vi "Serial_comm.vi"() -> ()   [LabVIEW 2022 SP3]
panel:
  in  "byte count":u32
  out "return count":u32
  out "read buffer":string
  in  "stop":bool
  in  "VISA resource name":refnum<visa-resource-name>
  # "This sets the number of digits displayed (1 digit = 1 byte) plus 2 bytes of terminating characters"
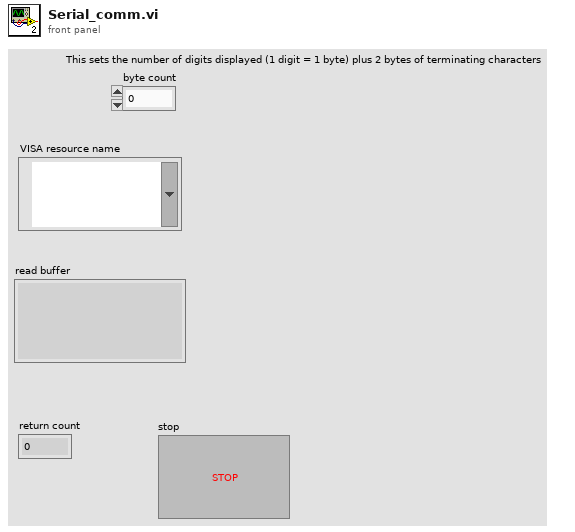
[diagram p1: front panel]
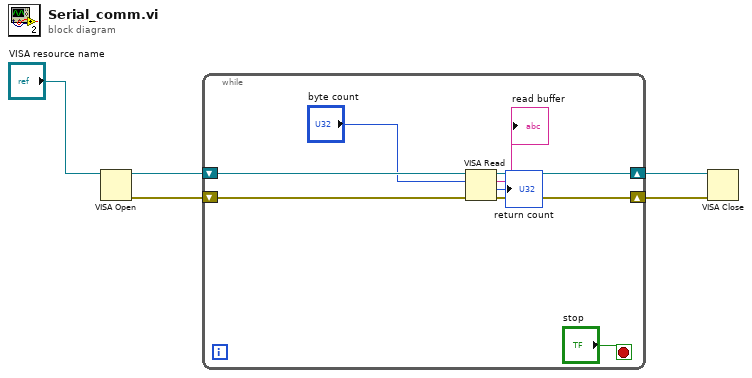
[diagram p0: block diagram]
diagram:
  n1 = VISA Open(VISA resource name="VISA resource name") -> (VISA resource name=w5:refnum<visa-resource-name>, error out=w3:errorcluster)  [unwired: 4 in]
  n2 = while {
    shift-right: [w13] -> w4
    shift-left: w5 -> [w7]
    shift-right: [w12] -> w2
    shift-left: w3 -> [w8]
    stop <- "stop" stop-if-true
    n3 = VISA Read(VISA resource name=w7, byte count="byte count", error in (no error)=w8) -> (VISA resource name out=w13:refnum<visa-resource-name>, read buffer=→"read buffer":string, return count=→"return count":u32, error out=w12:errorcluster)
  }
  n4 = VISA Close(VISA resource name=w4, error in (no error)=w2) -> ()  [unwired: 1 out]
